vi "Byte Buffer.Mapping.Create (Channel Pointer).vi"(8 "error in (no error)":errorcluster, 9 "data type":T1, 10 "buffer offset":i32, 11 "Channel Pointer":u64) -> (0 "error out":errorcluster, 2 "new buffer offset":i32, 3 "mapping":T2)   [LabVIEW 2016, in "VeriStand Data.lvlib" / "Byte Buffer.lvclass"]
uses:
  Byte Buffer.lvclass
  Byte Buffer.Mapping.ctl
  Typedefs/Typedefs.Data Types.ctl
  Utilities/Utilities.Sizeof.Scalar.vi
  VeriStand Data.lvlib
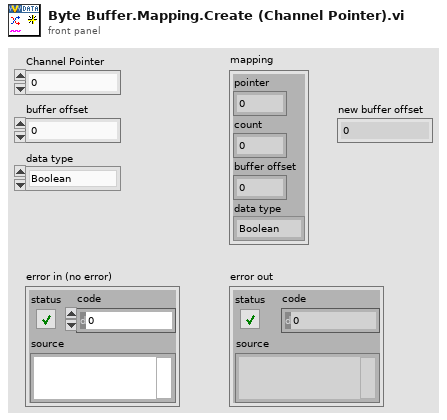
[diagram p1: front panel]
types:
  T1 = typedef "VeriStand Data.lvlib/Typedefs.Data Types.ctl" = enum16{"Boolean", "Single", "Double", "I8", "I16", "I32", "I64", "U8", "U16", "U32", "U64"}
  T2 = typedef "VeriStand Data.lvlib/Byte Buffer.lvclass/Byte Buffer.Mapping.ctl" = cluster{"pointer":u64, "count":i32, "buffer offset":i32, "data type":T1}
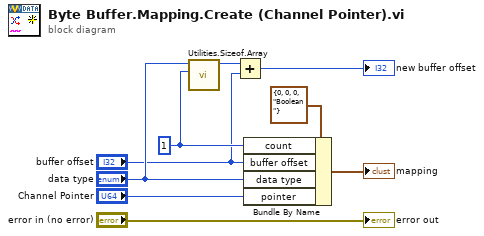
[diagram p0: block diagram]
diagram:
  w5 = 1 ("count")
  n1 = call "Utilities.Sizeof.Array.vi"("count"=w5, "data type"="data type") -> ("size"=w2:i32)  [unwired: 9 in]
  n2 = Add(x=w2, y="buffer offset") -> (x+y=→"new buffer offset":i32)
  n3 = Bundle By Name(cluster=T2 {"pointer"=0, "count"=0, "buffer offset"=0, "data type"=enum."Boolean"} ("mapping"), "count"=w5, "buffer offset"="buffer offset", "data type"="data type", "pointer"="Channel Pointer") -> (→"mapping":T2)
  "error out" <- "error in (no error)"
